vi "Check In Reference.vi"(8 "error in (no error)":errorcluster, 11 "Shape in":refnum<class "Shape.lvclass">) -> (0 "error out":errorcluster, 3 "Shape Reference":refnum<data-value>)   [LabVIEW 2015, in "LV Image Editor Framework.lvlib" / "Shape.lvclass"]
uses:
  Shape.lvclass
  Shape.lvclass/Shape.ctl
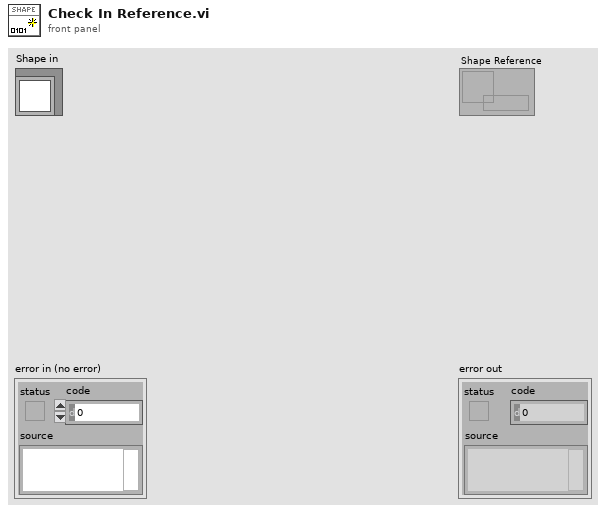
[diagram p1: front panel]
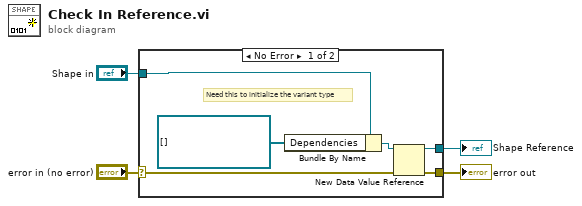
[diagram p0: block diagram]
diagram:
  n1 = case shown="No Error" "error in (no error)" {
    selector: "error in (no error)" -> [w9 w11]
    tunnel: [w8 w11] -> w3
    tunnel: [w10 _] -> w1
    tunnel: "Shape in" -> [w7 _]
    frame No Error {
      # "Need this to initialize the variant type"
      n2 = Bundle By Name(cluster=w7, "Dependencies"=refnum<data-value>[] [] ("data value reference")) -> (w6:refnum<class "Shape.lvclass">)
      n3 = New Data Value Reference(data value=w6, error in=w9) -> (data value reference=w10:refnum<data-value>, error out=w8:errorcluster)
    }
    frame Error {
    }
  }
  "error out" <- w3
  "Shape Reference" <- w1
